vi "GetGObjects_FP.vi"(8 "error in":errorcluster, 11 "VI Interpreter in":refnum<class "VI Interpreter.lvclass">) -> (0 "error out":errorcluster, 3 "VI Interpreter out":refnum<class "VI Interpreter.lvclass">)   [LabVIEW 2014, in "VI Interpreter.lvclass"]
uses:
  VI Interpreter.lvclass
  <vilib>/Utility/traverseref.llb/TRef TravTarget.ctl
  VI Interpreter.lvclass/VI Interpreter.ctl
  GObject/GObject.lvclass
  <vilib>/Utility/traverseref.llb/VI Scripting - Traverse.lvlib
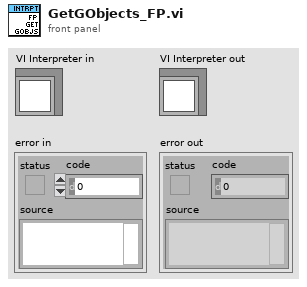
[diagram p1: front panel]
types:
  T1 = typedef "TRef TravTarget.ctl" = enum16{"FP", "BD", "Other"}
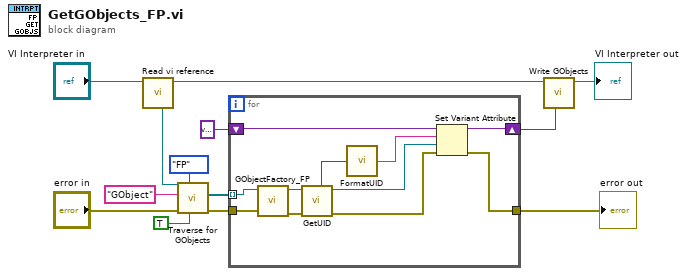
[diagram p0: block diagram]
diagram:
  n1 = call "Read vi reference.vi"("VI Interpreter in"="VI Interpreter in") -> ("VI Interpreter out"=w4:refnum<class "VI Interpreter.lvclass">, "vi reference"=w7:refnum<vi>)  [unwired: 7 in]
  n2 = call <vilib>:"Traverse for GObjects.vi"("Traverse Generated Code (F)"=TRUE, "Traverse Target"=TRef_TravTarget."FP", "error in (no error)"="error in", "Class Name"="GObject", "VI Refnum"=w7) -> ("error out"=w12:errorcluster, "References"=w10:refnum<vi>[])  [unwired: 3 in, 2 out]
  n3 = for {
    tunnel: w10 -> [w14] mode=indexing
    shift-right: [w24] -> w3
    shift-left: variant -> [w23]
    tunnel: w12 -> [w20]
    tunnel: [w22] -> w5
    n4 = call "GObjectFactory_FP.vi"("error in"=w20, "reference"=w14) -> ("error out"=w19:errorcluster, "GObject out"=w18:refnum<class "GObject.lvclass">)  [unwired: 8 in]
    n5 = call-dynamic "GetUID.vi"("error in"=w19, "GObject in"=w18) -> ("error out"=w15:errorcluster, "GObject out"=w16:refnum<class "GObject.lvclass">, "UID"=w17:i32)  [unwired: 5 in]
    n6 = call "FormatUID.vi"("UID"=w17) -> ("Name"=w21:string)
    n7 = Set Variant Attribute(Variant=w23, name=w21, value=w16, error in=w15) -> (Variant out=w24:variant, error out=w22:errorcluster)  [unwired: 1 out]
  }
  "error out" <- w5
  n8 = call "Write GObjects.vi"("GObjects"=w3, "VI Interpreter in"=w4) -> ("VI Interpreter out"=→"VI Interpreter out":refnum<class "VI Interpreter.lvclass">)  [unwired: 7 in]
